vi "Add Lib to Project.vi"() -> ()   [LabVIEW 2019]
uses:
  Source/VI Scripting Tools/Library/VI Scripting Tools.lvlib
panel:
  out "error out":errorcluster
  out "Build Specification Names":string[](array[string])
  in  "error in (no error)":errorcluster
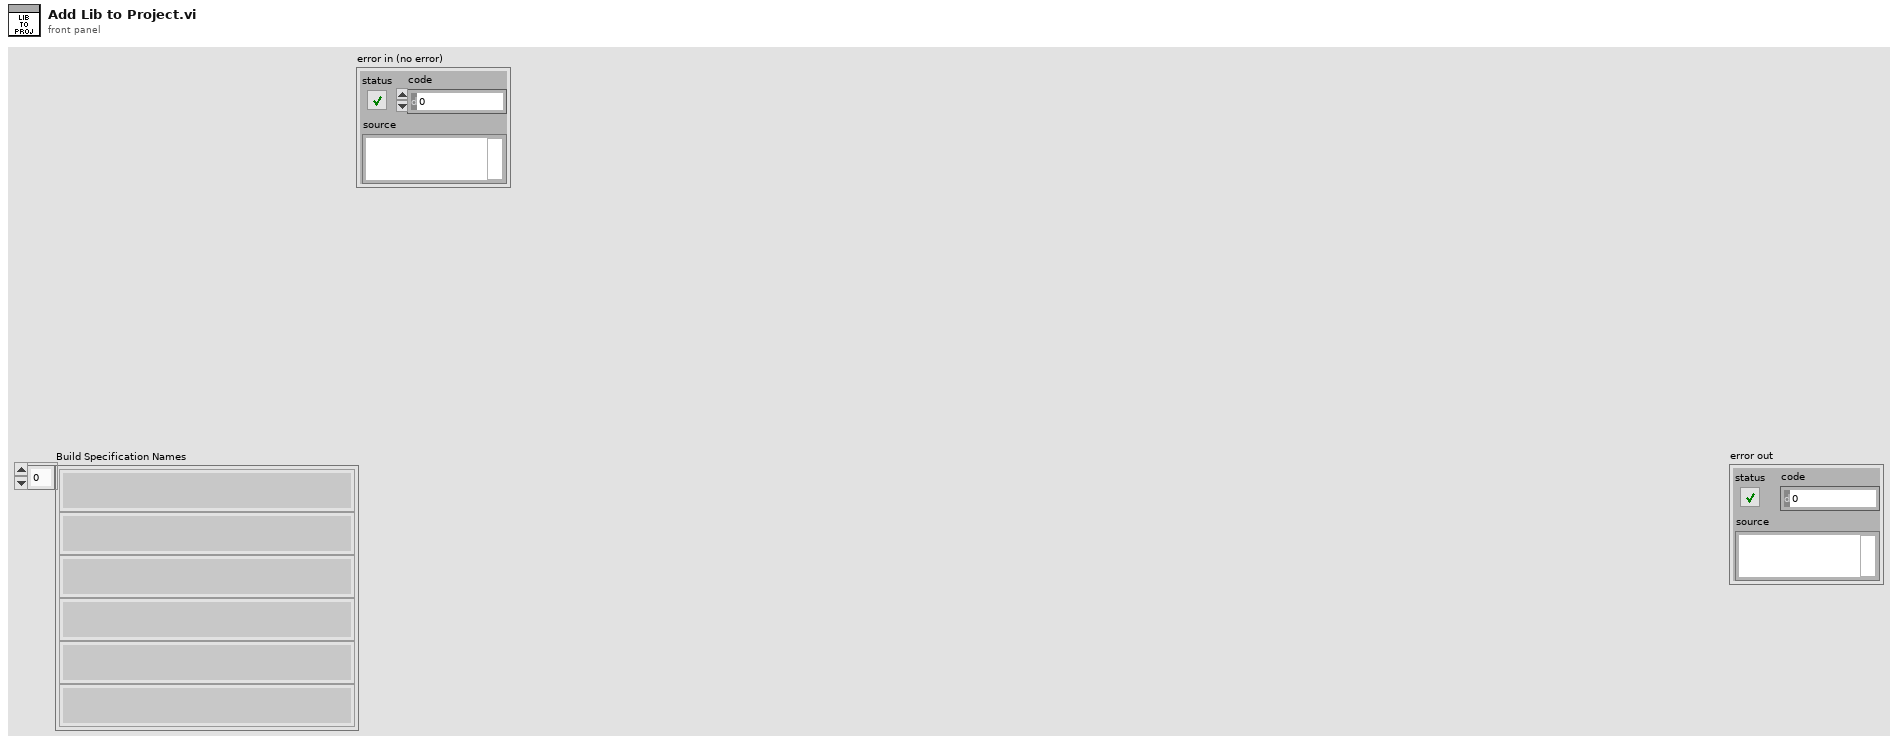
[diagram p1: front panel]
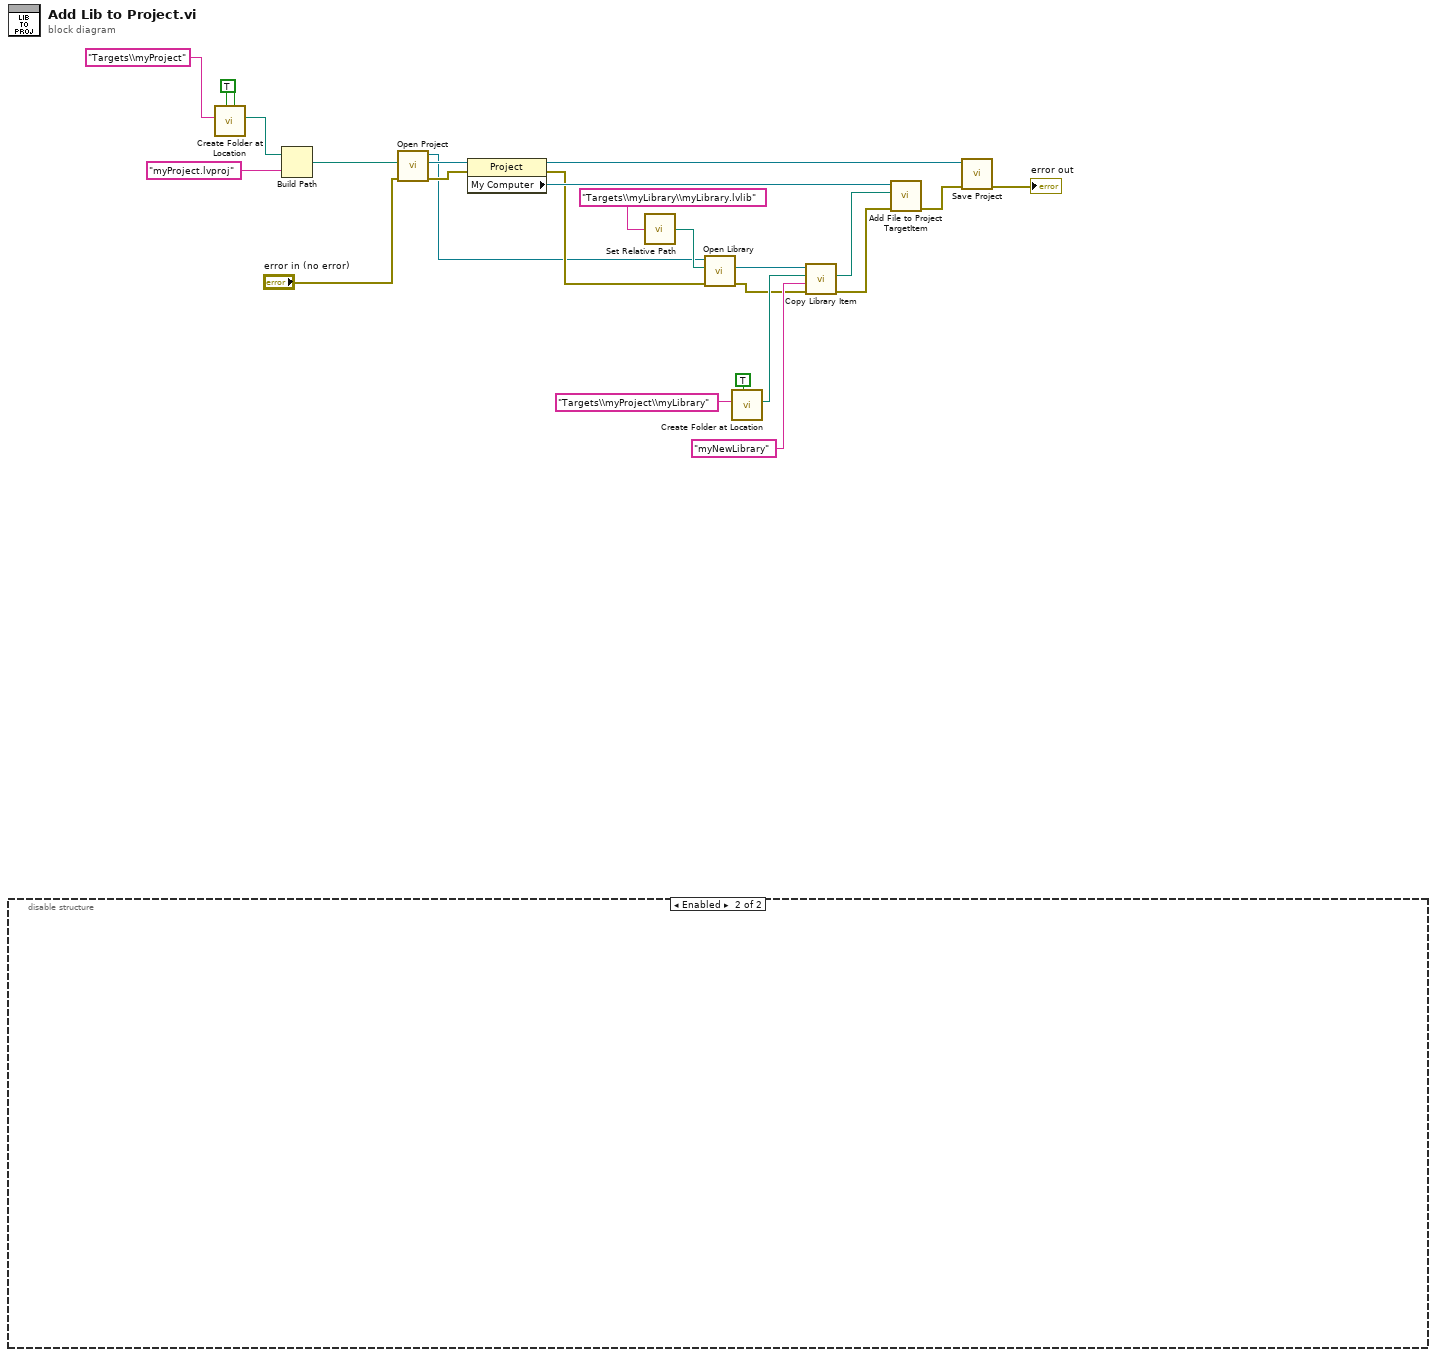
[diagram p0: block diagram]
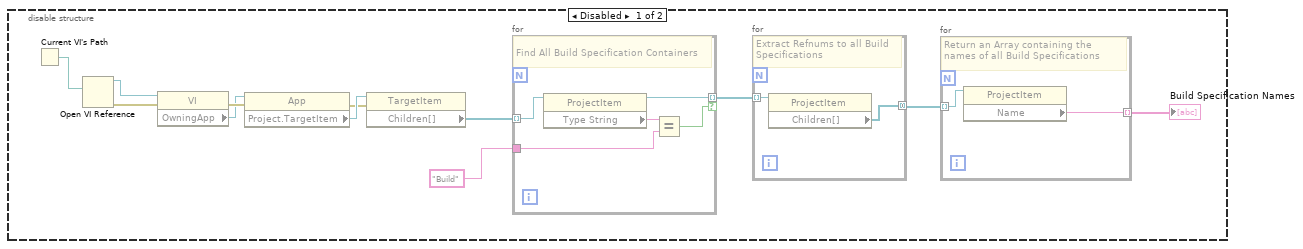
[diagram p2: hidden frame]
diagram:
  w23 = TRUE ("Use Relative")
  n1 = disable-structure shown="Enabled" {
    frame Disabled {
      n2 = Current VI's Path() -> (path=w27:path)
      n3 = Open VI Reference(vi path=w27) -> (vi reference=w28:refnum<vi>, error out=w29:errorcluster)  [unwired: 5 in]
      n4 = property class="VI"(reference=w28, error in=w29) -> (error out=w35:errorcluster, "OwningApp"=w30:refnum<vi>)  [unwired: 1 out]
      n5 = property class="App"(reference=w30, error in=w35) -> (error out=w31:errorcluster, "Project.TargetItem"=w32:refnum<vi>)  [unwired: 1 out]
      n6 = property class="TargetItem"(reference=w32, error in=w31) -> ("Children[]"=w33:refnum<vi>[])  [unwired: 2 out]
      n7 = for {
        tunnel: w33 -> [w45] mode=indexing
        tunnel: [w43] -> w34 mode=indexing if=w42
        tunnel: "Build" ("y") -> [w41]
        # "Find All Build Specification Containers"
        n8 = property class="ProjectItem"(reference=w45) -> (reference out=w43:refnum<vi>, "Type String"=w44:string)  [unwired: 1 in, 1 out]
        n9 = Equal?(x=w44, y=w41) -> (x = y?=w42:bool)
      }
      n10 = for {
        tunnel: w34 -> [w40] mode=indexing
        tunnel: [w39] -> w25 mode=concatenating
        # "Extract Refnums to all Build Specifications"
        n11 = property class="ProjectItem"(reference=w40) -> ("Children[]"=w39:refnum<vi>[])  [unwired: 1 in, 2 out]
      }
      n12 = for {
        tunnel: w25 -> [w38] mode=indexing
        tunnel: [w37] -> w26 mode=indexing
        # "Return an Array containing the names of all Build Specifications"
        n13 = property class="ProjectItem"(reference=w38) -> ("Name"=w37:string)  [unwired: 1 in, 2 out]
      }
      "Build Specification Names" <- w26
    }
    frame Enabled {
    }
  }
  n14 = call "Create Folder at Location.vi"("Override existing"=w23, "Use Relative"=w23, "Path"="Targets\\myProject") -> ("Full path out"=w15:path)  [unwired: 7 in, 1 out]
  n15 = Build Path(base path=w15, name or relative path="myProject.lvproj") -> (appended path=w22:path)
  n16 = call "Open Project.vi"("error in (no error)"="error in (no error)", "Project Path in"=w22) -> ("error out"=w16:errorcluster, "Project out"=w19:refnum<vi>, "Application out"=w1:refnum<vi>)  [unwired: 7 in]
  n17 = property class="Project"(reference=w19, error in=w16) -> (reference out=w4:refnum<vi>, error out=w9:errorcluster, "My Computer"=w18:refnum<vi>)
  n18 = call "Set Relative Path.vi"("App Relative Path"="Targets\\myLibrary\\myLibrary.lvlib") -> ("Full Path"=w8:path)
  n19 = call "Open Library.vi"("error in (no error)"=w9, "Full Path"=w8, "Application in"=w1) -> ("error out"=w7:errorcluster, "Library out"=w6:refnum<vi>)  [unwired: 6 in, 1 out]
  n20 = call "Create Folder at Location.vi"("Use Relative"=TRUE, "Path"="Targets\\myProject\\myLibrary") -> ("Full path out"=w12:path)  [unwired: 8 in, 1 out]
  n21 = call "Copy Library Item.vi"("error in (no error)"=w7, "Copy Name"="myNewLibrary" ("name or relative path"), "Copy location"=w12, "Library in"=w6) -> ("error out"=w5:errorcluster, "New Lib Path"=w10:path)  [unwired: 5 in, 1 out]
  n22 = call "Add File to Project TargetItem.vi"("error in (no error)"=w5, "New File Location"=w10, "Project TargetItem in"=w18) -> ("error out"=w3:errorcluster)  [unwired: 6 in, 2 out]
  n23 = call "Save Project.vi"("error in (no error)"=w3, "Project in"=w4) -> ("error out"=→"error out":errorcluster)  [unwired: 8 in, 1 out]
